vi "Test HDW.vi"(8 "error in (no error)":errorcluster, 11 "Mag Lab Hardware in":refnum<class "Mag Lab Hardware.lvclass">) -> (0 "error out":errorcluster, 3 "Mag Lab Hardware out":refnum<class "Mag Lab Hardware.lvclass">)   [LabVIEW 2015]
uses:
  Mag Lab Hardware.lvclass
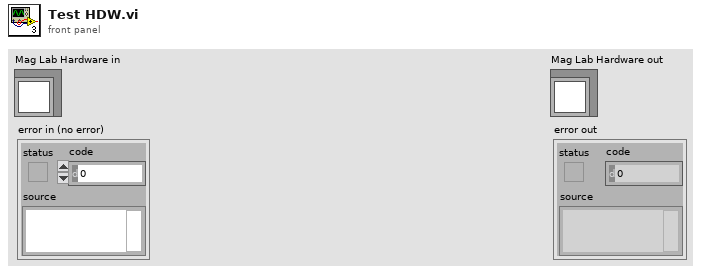
[diagram p1: front panel]
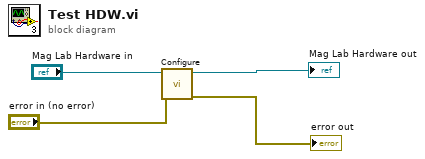
[diagram p0: block diagram]
diagram:
  n1 = call-dynamic "Configure.vi"("error in (no error)"="error in (no error)", "Mag Lab Root in"="Mag Lab Hardware in") -> ("error out"=→"error out":errorcluster, "Mag Lab Root out"=→"Mag Lab Hardware out":refnum<class "Mag Lab Hardware.lvclass">)  [unwired: 8 in]
